vi "SLSC Scripting Constants.vi"() -> ()   [LabVIEW 2017, in "SLSC Switch Scripting.lvlib"]
doc: "Use this Global VI to access the GUIDs assigned to the page resources of the Custom Device."
uses:
  SLSC Switch Scripting.lvlib
panel:
  in  "Tab Control":T1(tab)=enum."SLSC Switch Constants"
  in  "SLSC Switch:CD:GUID":string="5e47c8de-3ec6-490b-8897-5526d4aea756"
  in  "RAF:CD:GUID":string="4e591626-626d-4903-9a6e-1f2a7b879f4d"
  in  "SLSC Sw:Prop:Model":string="Model"
  in  "SLSC Sw:Prop:Capabilities Version":string="Capabilities Version"
  in  "SLSC Sw:Prop:Resource":string="Resource "
  in  "SLSC Sw:Prop:Topology":string="Topology "
  in  "SLSC Sw:Prop:Capabilities":string="Capabilities "
  in  "SLSC Sw:Endpoint Section":string="Endpoint Configuration"
  in  "Compiled.Settings":string="Compiled.Settings"
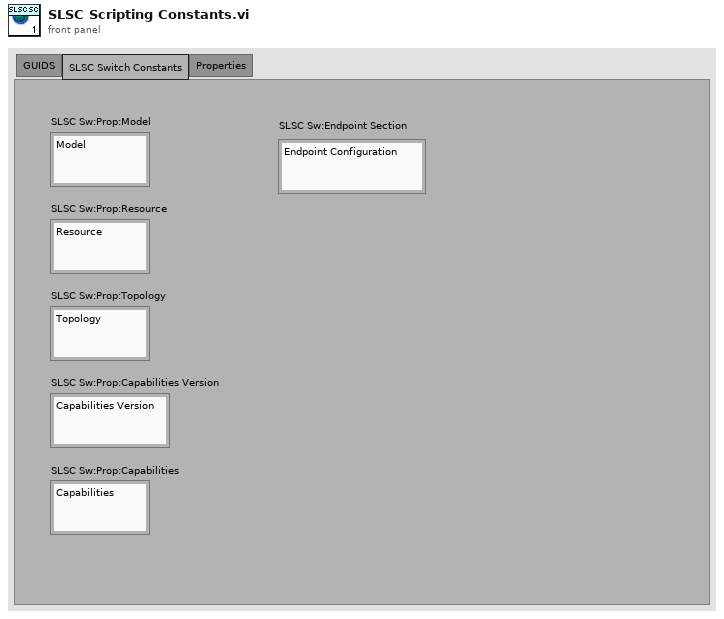
[diagram p1: front panel]
types:
  T1 = enum32{"GUIDS", "SLSC Switch Constants", "Properties"}
diagram:
